vi "Bind Terminal.vi"(6 "Value Changes Only? (F)":bool, 7 "Use Label Text (F=Use Caption)":bool, 8 "error in (no error)":errorcluster, 9 "Topic Name (Use Control Text)":string, 10 "Ctl Refnum":refnum<vi>, 11 "IObserver in":refnum<class "IObserver.lvclass">) -> (0 "error out":errorcluster, 3 "IObserver out":refnum<class "IObserver.lvclass">)   [LabVIEW 2015, in "IObserver.lvlib" / "IObserver.lvclass"]
uses:
  IObserver.lvclass
  <vilib>/ActorFramework/Actor/Actor.lvclass/Actor.ctl
  <vilib>/ActorFramework/Message Enqueuer/Message Enqueuer.lvclass/Message Enqueuer.ctl
  IMediator/SubscriptionPolicy/SubscriptionPolicy.lvclass/SubscriptionPolicy.ctl
  IObserver Messages/Subscribe Msg/Subscribe Msg.lvclass/Subscribe Msg.ctl
  <vilib>/ActorFramework/Message Enqueuer/Init from Existing Queue.vi
  <vilib>/ActorFramework/Message Enqueuer/Enqueue.vi
  <vilib>/ActorFramework/Message Priority Queue/Priority Enqueue.vi
  <vilib>/ActorFramework/Message Enqueuer/Message Enqueuer.lvclass
  IMediator/SubscriptionPolicy/SubscriptionPolicy.lvclass
  IObserver Messages/Subscribe Msg/Subscribe Msg.lvclass
  IMediator/SubscriptionRequest/SubscriptionRequest.lvclass
  <vilib>/ActorFramework/Actor/Actor.lvclass
  Mediator/Transport/TerminalBinding/TerminalBinding.lvclass
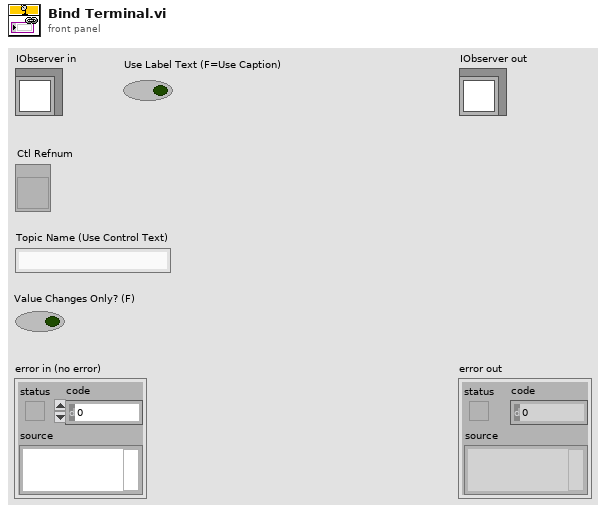
[diagram p1: front panel]
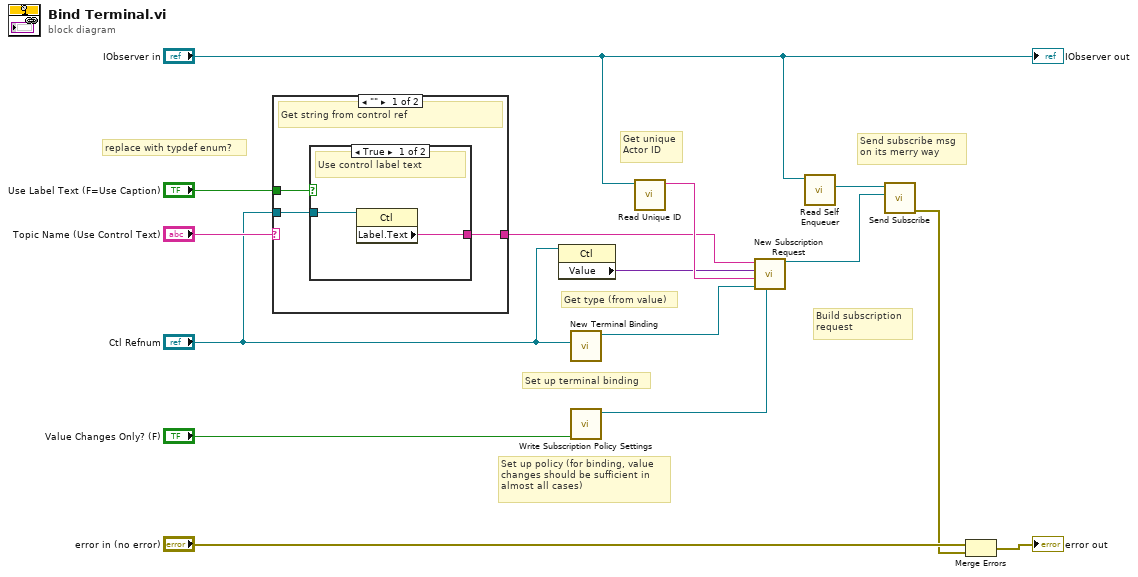
[diagram p0: block diagram]
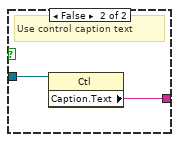
[diagram p2: hidden frame]
diagram:
  # "Set up policy (for binding, value\nchanges should be sufficient in\nalmost all cases)"
  # "replace with typdef enum?"
  # "Send subscribe msg\non its merry way"
  # "Build subscription\nrequest"
  # "Get unique\nActor ID"
  # "Get type (from value)"
  # "Set up terminal binding"
  n1 = case shown="\"\"" "Topic Name (Use Control Text)" {
    selector: "Topic Name (Use Control Text)" -> [_ w23]
    tunnel: [w16 w23] -> w4
    tunnel: "Use Label Text (F=Use Caption)" -> [w18 _]
    tunnel: "Ctl Refnum" -> [w17 _]
    frame "" {
      # "Get string from control ref"
      n2 = case shown="True" w18 {
        tunnel: w17 -> [w20 w22]
        tunnel: [w19 w21] -> w16
        frame True {
          # "Use control label text"
          n3 = property class="Ctl"(reference=w20) -> ("Label.Text"=w19:string)  [unwired: 1 in, 2 out]
        }
        frame False {
          # "Use control caption text"
          n4 = property class="Ctl"(reference=w22) -> ("Caption.Text"=w21:string)  [unwired: 1 in, 2 out]
        }
      }
    }
    frame Default {
      # "Use string wired to input terminal"
    }
  }
  n5 = property class="Ctl"(reference="Ctl Refnum") -> ("Value"=w12:variant)  [unwired: 1 in, 2 out]
  n6 = call "New Terminal Binding.vi"("Ctl Refnum"="Ctl Refnum") -> ("TerminalBinding out"=w14:refnum<class "TerminalBinding.lvclass">)  [unwired: 9 in, 1 out]
  n7 = call "Write Subscription Policy Settings.vi"("Value Changes Only? (F)"="Value Changes Only? (F)") -> ("SubscriptionPolicy out"=w2:refnum<class "SubscriptionPolicy.lvclass">)  [unwired: 10 in]
  n8 = call "Read Unique ID.vi"("IObserver In"="IObserver in") -> ("Unique ID"=w13:string)  [unwired: 10 in]
  n9 = call "New Subscription Request.vi"("SubscriptionPolicy"=w2, "Transport"=w14, "Unique Subscriber ID"=w13, "Type"=w12, "Topic Name"=w4) -> ("SubscriptionRequest out"=w9:refnum<class "SubscriptionRequest.lvclass">)  [unwired: 6 in]
  n10 = call <vilib>:"Read Self Enqueuer.vi"("Actor"="IObserver in") -> ("Self Enqueuer"=w10:refnum<class "Message Enqueuer.lvclass">)  [unwired: 10 in]
  n11 = call "Send Subscribe.vi"("SubscriptionRequest"=w9, "Message Enqueuer"=w10) -> ("error out"=w7:errorcluster)  [unwired: 8 in, 1 out]
  n12 = Merge Errors("error in (no error)", w7) -> (→"error out":errorcluster)
  "IObserver out" <- "IObserver in"
